vi "PTScanner.set state.vi"(0 "i ref in":refnum<vi>, 2 "state":string, 5 "error in (no error)":errorcluster) -> (14 "i ref out":refnum<vi>, 19 "error out":errorcluster)   [LabVIEW 2014, in "PTScanner.lvlib"]
uses:
  PTScanner.lvlib
  CS_Core/BaseSM/BaseSM.lvlib
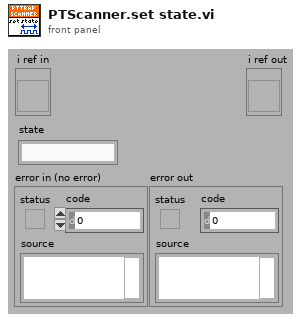
[diagram p1: front panel]
types:
  T1 = typedef "BaseSM.lvlib/BaseSM.i attribute.ctl" = cluster{"stateError":i32, "stateStatus":string, "stateQuality":T2, "ProcStateRef":refnum<vi>, "thread ref":refnum<vi>, "actState":string, "reqState":string, "SMQueue":refnum<queue>, "stateErrorID":i32, "stateStatusID":i32}
  T2 = typedef "BaseSM.lvlib/BaseSM.stateQuality.ctl" = i16
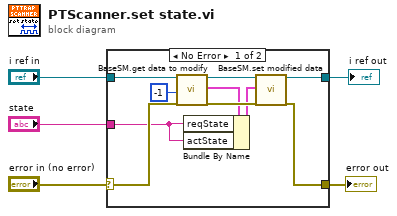
[diagram p0: block diagram]
diagram:
  n1 = case shown="No Error" "error in (no error)" {
    selector: "error in (no error)" -> [w7 w16]
    tunnel: "i ref in" -> [w14 w17]
    tunnel: [w13 w16] -> w4
    tunnel: [w12 w17] -> w3
    tunnel: "state" -> [w6 _]
    frame No Error {
      n2 = call "BaseSM.get data to modify.vi"("i ref in"=w14, "ms timeout (10000)"=-1, "error in (no error)"=w7) -> ("i ref out"=w11:refnum<vi>, "i attribute"=w9:T1, "error out"=w15:errorcluster)  [unwired: 13 in, 1 out]
      n3 = Bundle By Name(cluster=w9, "reqState"=w6, "actState"=w6) -> (w8:T1)
      n4 = call "BaseSM.set modified data.vi"("i ref in"=w11, "i attribute"=w8, "error in (no error)"=w15) -> ("i ref out"=w12:refnum<vi>, "error out"=w13:errorcluster)  [unwired: 15 in]
    }
    frame Error {
    }
  }
  "error out" <- w4
  "i ref out" <- w3
